vi "Autonomous Independent.vi"() -> ()   [LabVIEW 2020]
doc: "This VI is called when autonomous begins, and will automatically be terminated when autonomous ends. You can carry out timed or sensor driven robot movement independently without needing to return to the caller."
uses:
  <vilib>/Rock Robotics/WPI/RobotDrive/WPI_RobotDriveArcadeDrive_Standard(NoSaturation).vi
  <vilib>/Rock Robotics/Network Tables/NT Write Numeric Array.vi
  <vilib>/Rock Robotics/WPI/ThirdParty/Phoenix-LabVIEW/Motor Controller/Controls/CTRE_Phoenix_MotorControl_ControlMode.ctl
  <vilib>/Rock Robotics/WPI/ThirdParty/Phoenix-LabVIEW/CANCoder/Get/CTRE_Phoenix_CANcoder_GetSensorData.vi
  <vilib>/Rock Robotics/WPI/ThirdParty/Phoenix-LabVIEW/Motor Controller/Get/CTRE_Phoenix_MotorController_GetSelectedSensorData.vi
  <vilib>/Rock Robotics/WPI/Solenoid/WPI_SolenoidValue.ctl
  <vilib>/Rock Robotics/WPI/Solenoid/WPI_SolenoidSetEnum.vi
  <vilib>/Rock Robotics/Network Tables/NT Read String.vi
panel:
  out "Talon Encoder Values 2":i32
  out "Arm Tellescope position":dbl format="%#_13g"
  out "Angle Position":dbl format="%#_13g"
  out "Talon Encoder Values":i32=45
  out "Current Movement, for debugging":T1 {"Y Joystick Value" scale=1.0..-1.0; "X Joystick Value" scale=-1.0..1.0}
  in  "Array of robot movements":T2(array[cluster])=[{"X Joystick Value"=0.39393939393939403, "Y Joystick Value"=0.0, "Delay (sec)"=1.0, "Movement Name"="turn"}, {"X Joystick Value"=-0.3737373737373737, "Y Joystick Value"=0.0, "Delay (sec)"=1.0, "Movement Name"="turn back"}] {"Y Joystick Value" scale=1.0..-1.0; "X Joystick Value" scale=-1.0..1.0}
  # "Be sure to right-click and choose Data Operations>>Make Current Value default if you want to save the array values with the VI"
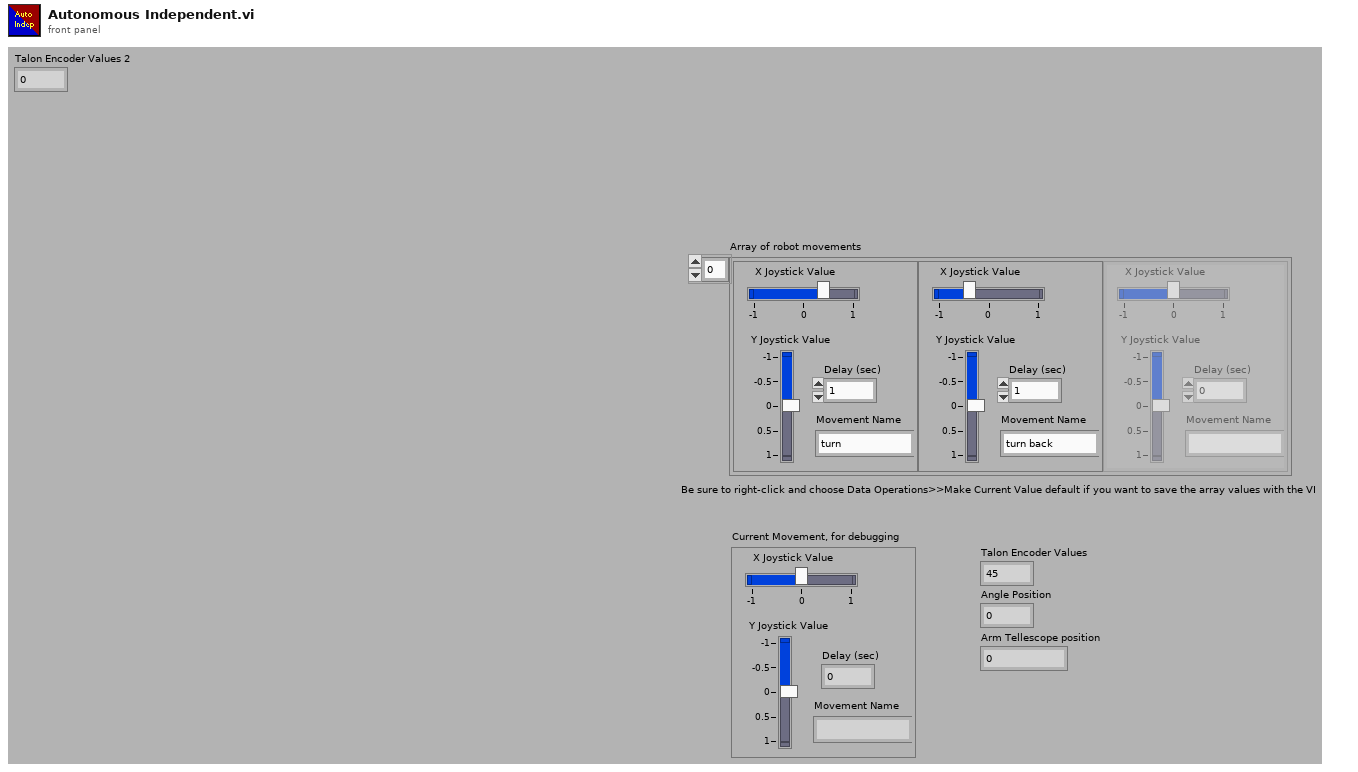
[diagram p1: front panel]
types:
  T1 = cluster{"X Joystick Value":dbl, "Y Joystick Value":dbl, "Delay (sec)":dbl, "Movement Name":string}
  T2 = cluster{"X Joystick Value":dbl, "Y Joystick Value":dbl, "Delay (sec)":dbl, "Movement Name":string}[]
  T3 = typedef "WPI_JoystickDevRef.ctl" = cluster{"Device":T4}
  T4 = typedef "WPI_JoystickDeviceEnum.ctl" = enum16{"USB 0", "USB 1", "USB 2", "USB 3", "USB 4", "USB 5"}
  T5 = typedef "WPI_SolenoidValue.ctl" = enum16{"Off", "On", "Forward", "Reverse"}
  T6 = typedef "WPI_MotorControlDeviceRef.ctl" = cluster{"DeviceStatus":errorcluster, "Type":T7, "PWM":cluster{"PWM Channel":T8, "DeadBand":T9}, "CAN":cluster{"Device Number":u8, "SetOutput VI Ref":variant, "GetOutput VI Ref":variant, "Enable VI Ref":variant, "Disable VI Ref":variant, "Data":variant}, "Invert":bool, "DIO PWM":cluster{"PWM \"Enable\" Channel":T8, "DIOChannel":T10, "PWM Rate":dbl}}
  T7 = typedef "WPI_MotorControlType.ctl" = enum16{"PWM", "CAN", "DIO PWM"}
  T8 = typedef "FPGA_DIOPWMChannel.ctl" = enum8{"PWM 0", "PWM 1", "PWM 2", "PWM 3", "PWM 4", "PWM 5", "PWM 6", "PWM 7", "PWM 8", "PWM 9", "PWM MXP 0", "PWM MXP 1", "PWM MXP 2", "PWM MXP 3", "PWM MXP 4", "PWM MXP 5", "PWM MXP 6", "PWM MXP 7", "PWM MXP 8", "PWM MXP 9", "Invalid"}
  T9 = typedef "WPI_PWMDeadband.ctl" = cluster{"Name":string, "maxPositivePwm":i32, "minPositivePwm":i32, "centerPwm":i32, "maxNegativePwm":i32, "minNegativePwm":i32, "angularRange":u16}
  T10 = typedef "FPGA_DIOChannel.ctl" = enum8{"DIO 0", "DIO 1", "DIO 2", "DIO 3", "DIO 4", "DIO 5", "DIO 6", "DIO 7", "DIO 8", "DIO 9", "DIO MXP 0", "DIO MXP 1", "DIO MXP 2", "DIO MXP 3", "DIO MXP 4", "DIO MXP 5", "DIO MXP 6", "DIO MXP 7", "DIO MXP 8", "DIO MXP 9", "DIO MXP 10", "DIO MXP 11", "DIO MXP 12", "DIO MXP 13", "DIO MXP 14", "DIO MXP 15", "SPI Port CS1", "SPI Port CS2", "SPI Port CS3", "SPI Port MISO", "SPI Port MOSI", "Invalid"}
  T11 = typedef "WPI_RobotDriveDevRef.ctl" = cluster{"DevStatus":errorcluster, "Motors[]":T6[], "Square Inputs":bool, "Max Output":dbl}
  T12 = typedef "CTRE_Phoenix_CANcoder_DeviceRef.ctl" = cluster{"DeviceStatus":errorcluster, "Device Number":u8, "Handle":u64, "UsageFrame":u32, "Library Path":path}
  T13 = typedef "WPI_SolenoidDevRef.ctl" = cluster{"DevStatus":errorcluster, "Pneumatics Control Module":u8, "Forward Solenoid Channel":T14, "Reverse Solenoid Channel":T14}
  T14 = typedef "WPI_SolenoidChannel.ctl" = enum8{"Solenoid 0", "Solenoid 1", "Solenoid 2", "Solenoid 3", "Solenoid 4", "Solenoid 5", "Solenoid 6", "Solenoid 7", "Solenoid 8", "Solenoid 9", "Solenoid 10", "Solenoid 11", "Solenoid 12", "Solenoid 13", "Solenoid 14", "Solenoid 15", "Invalid"}
  T15 = typedef "CTRE_Phoenix_MotorControl_ControlMode.ctl" = u16
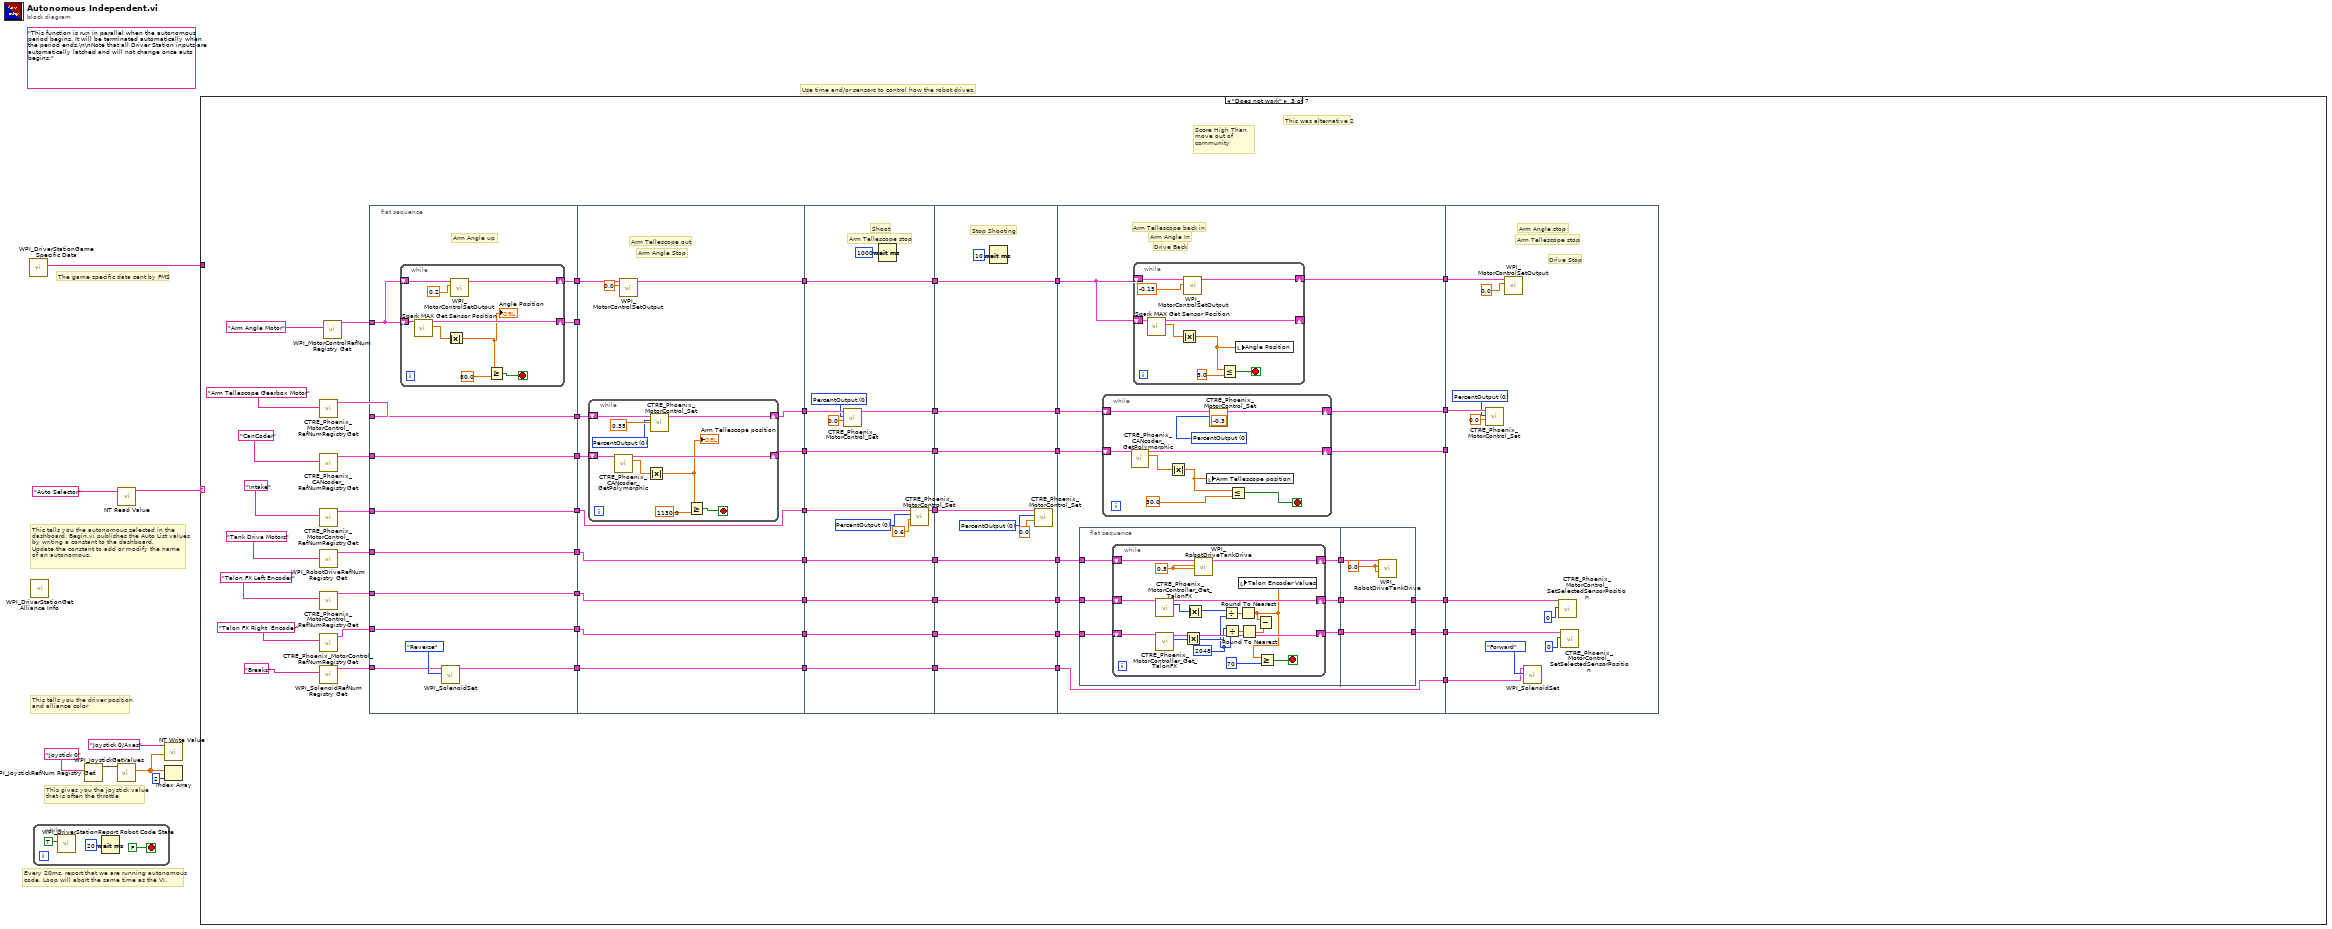
[diagram p0: block diagram]
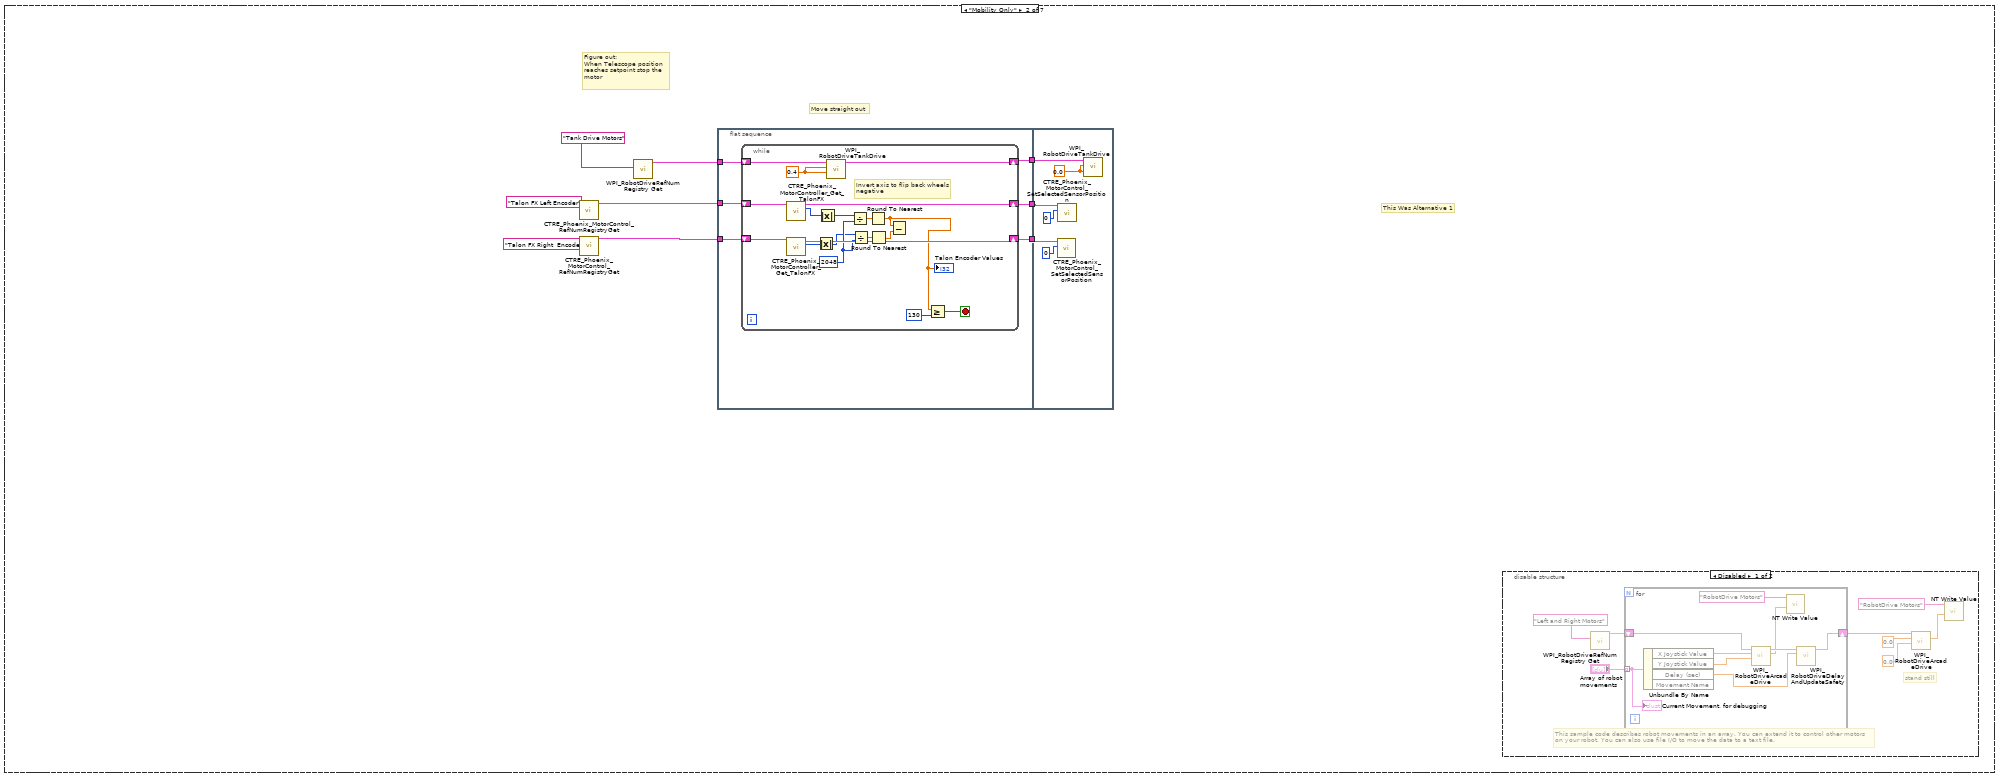
[diagram p3: hidden frame]
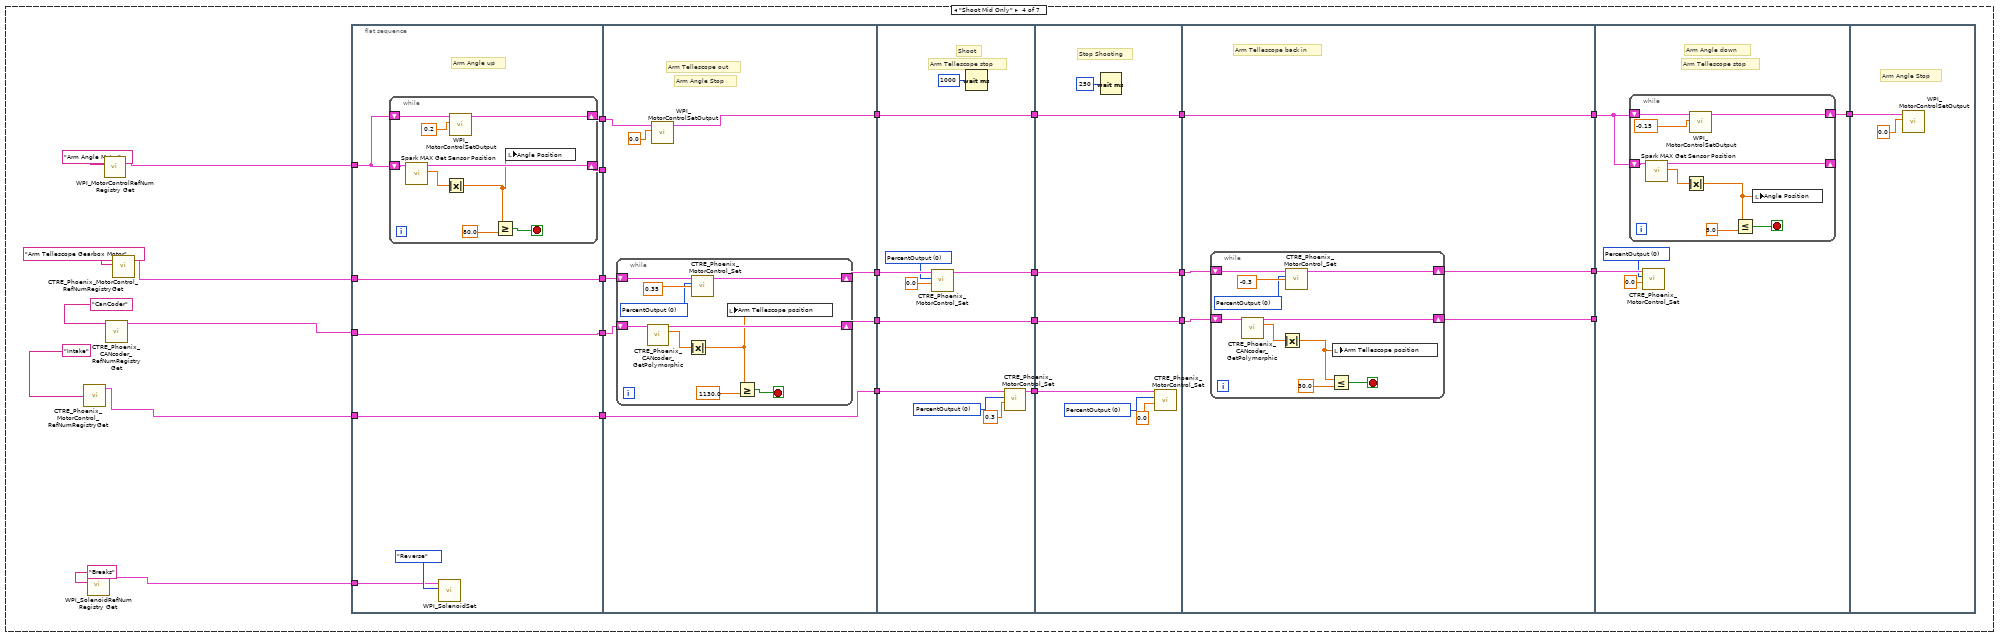
[diagram p5: hidden frame]
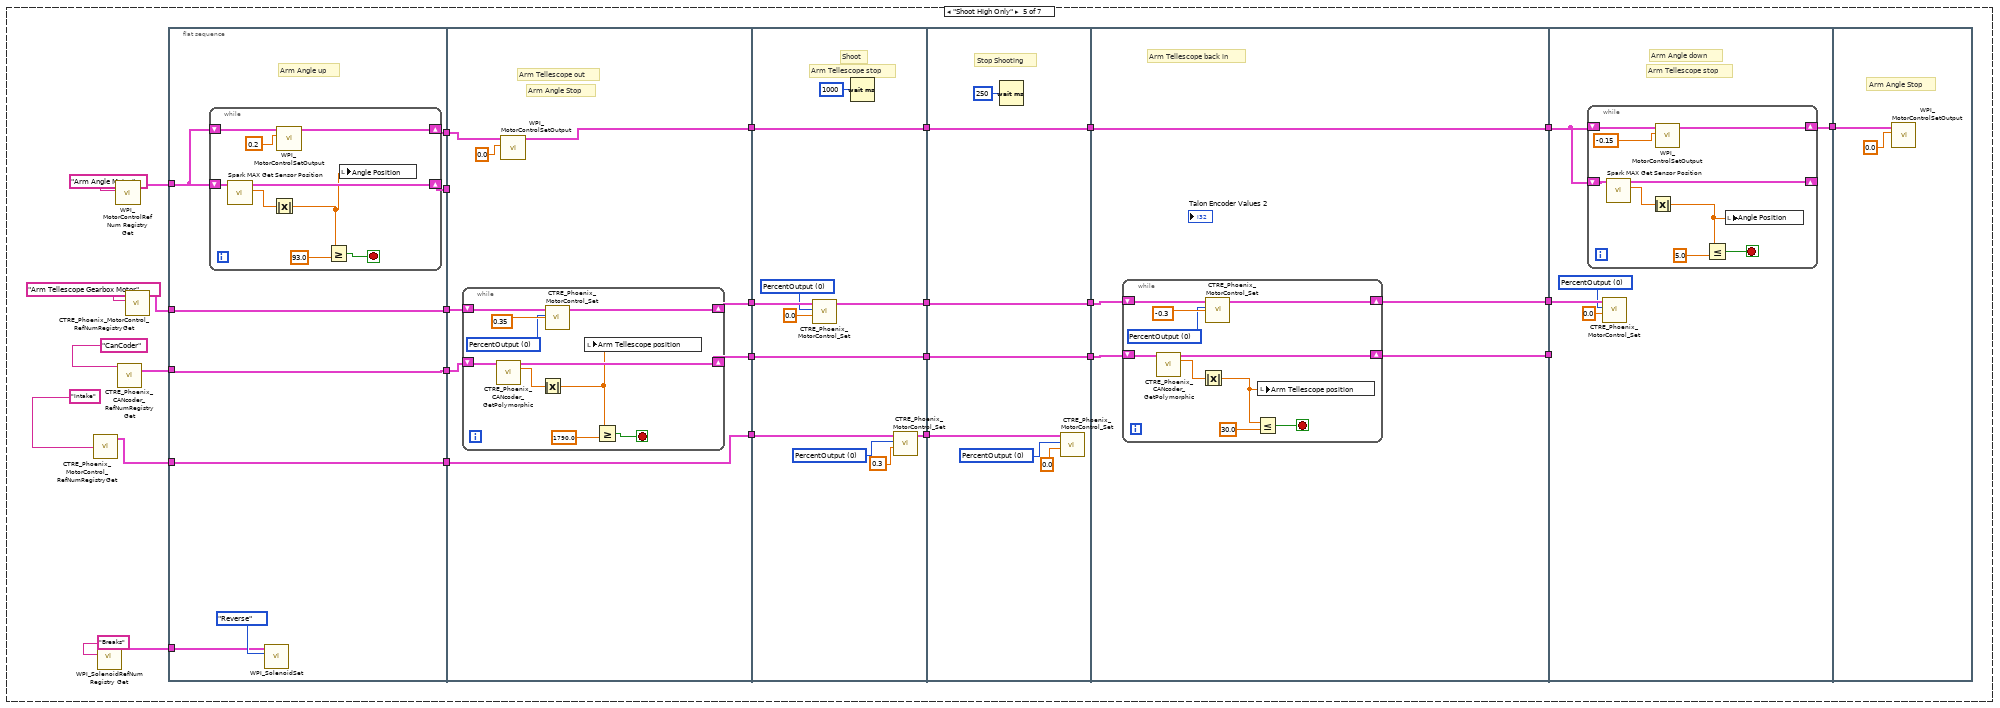
[diagram p6: hidden frame]
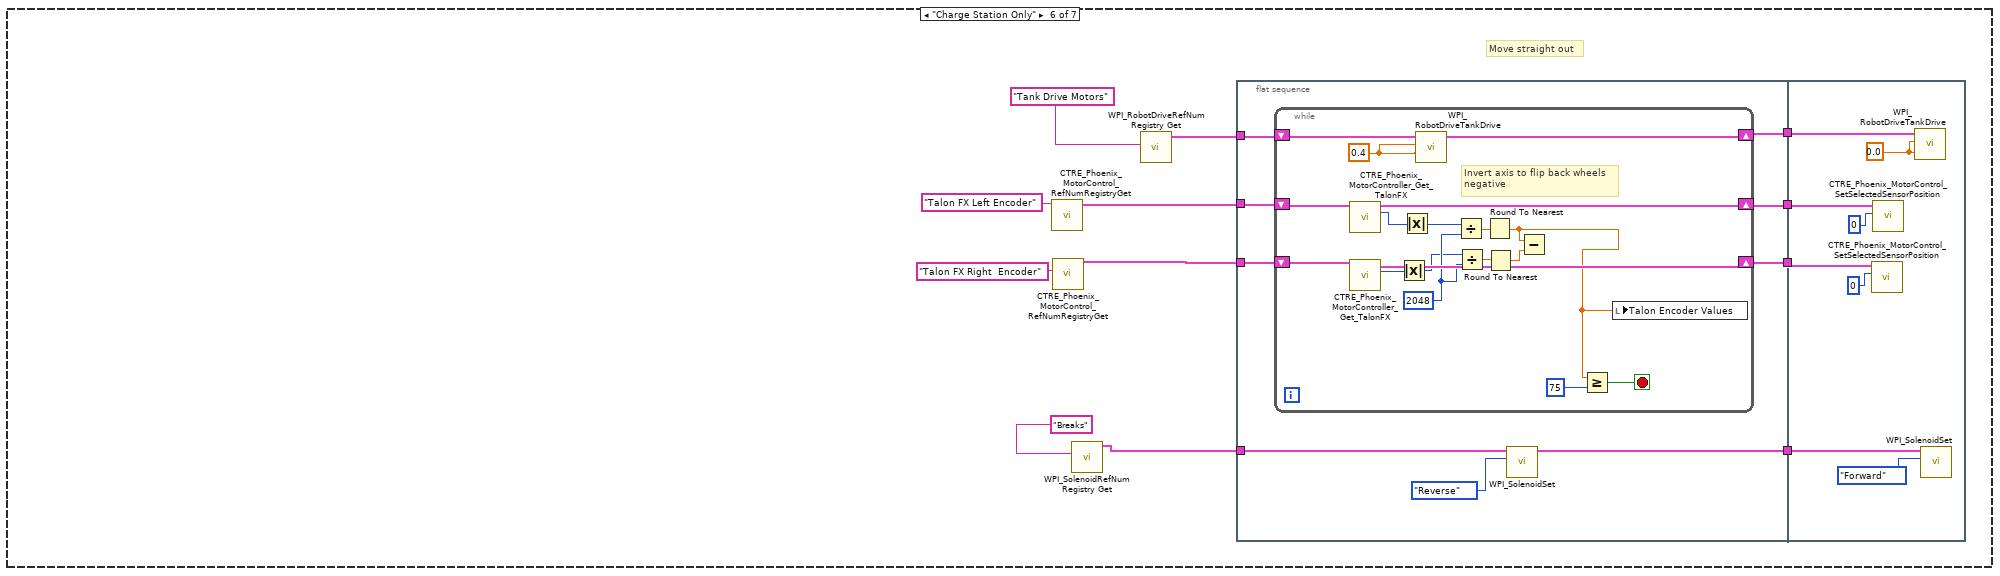
[diagram p7: hidden frame]
diagram:
  (unwired) "This function is run in parallel when the autonomous period begins. It will be terminated automatically when the period ends.\n\nNote that all Driver Station inputs are automatically latched and will not change once auto begins."
  # "The game specific data sent by FMS"
  # "This tells you the autonomous selected in the \ndashboard. Begin.vi publishes the Auto List values\nby writing a constant to the dashboard.\nUpdate the constant to add or modify the name\nof an autonomous."
  # "Every 20ms, report that we are running autonomous\ncode. Loop will abort the same time as the VI."
  # "This gives you the joystick value\nthat is often the throttle"
  # "Use time and/or sensors to control how the robot drives."
  # "This tells you the driver position\nand alliance color"
  n1 = call <vilib>:"WPI_DriverStationGame Specific Data.vi"() -> ("Game Specific Data"=w1:string)  [unwired: 11 in]
  n2 = call <vilib>:"WPI_DriverStationGet Alliance Info.vi"() -> ()  [unwired: 12 out]
  n3 = while {
    stop <- FALSE stop-if-true
    n4 = call <vilib>:"WPI_DriverStationReport Robot Code State.vi"("Autonomous"=TRUE) -> ()  [unwired: 10 in, 1 out]
    n5 = Wait (ms)(milliseconds to wait=u32 20) -> ()  [unwired: 1 out]
  }
  n6 = call <vilib>:"WPI_JoystickRefNum Registry Get.vi"("refnum name"="Joystick 0") -> ("JoystickDevRef"=w7:T3)  [unwired: 1 in, 9 out]
  n7 = call <vilib>:"WPI_JoystickGetValues.vi"("JoystickDevRef"=w7) -> ("Axes"=w3:dbl[])  [unwired: 6 in, 4 out]
  n8 = call-poly <vilib>:"NT Read Value.vi"("name"="Auto Selector" ("Name")) -> ("value"=w4:string)  [unwired: 8 in, 2 out]
  n9 = call-poly <vilib>:"NT Write Value.vi"("value"=w3, "name"="Joystick 0/Axes" ("Name")) -> ()  [unwired: 9 in, 1 out]
  n10 = Index Array(array=w3, index=2) -> ()  [unwired: 1 out]
  n11 = case shown="\"Does not work\"" w4 {
    tunnel: w1 -> [_ _ _ _ _ _ _]
    frame Default {
      # "You can put your main auto here, or you can right-click on the case and make any\nother frame be the default case."
      # "This is the frame that will execute if no selection is made, or if it is not recognized"
    }
    frame "Mobility Only" {
      # "Move straight out"
      # "This Was Alternative 1"
      # "Figure out:\nWhen Telescope position  \nreaches setpoint stop the \nmotor"
      n12 = call <vilib>:"CTRE_Phoenix_MotorControl_RefNumRegistryGet.vi"("refnum name"="Talon FX Left Encoder") -> ("PhoenixMotorControlDevRef"=w12:T6)  [unwired: 9 in, 1 out]
      n13 = call <vilib>:"CTRE_Phoenix_MotorControl_RefNumRegistryGet.vi"("refnum name"="Talon FX Right  Encoder") -> ("PhoenixMotorControlDevRef"=w13:T6)  [unwired: 9 in, 1 out]
      n14 = call <vilib>:"WPI_RobotDriveRefNum Registry Get.vi"("refnum name"="Tank Drive Motors") -> ("RobotDriveDevRef"=w16:T11)  [unwired: 9 in, 1 out]
      n15 = flat-sequence {
        tunnel: w16 -> [w43]
        tunnel: [w42] -> w20
        tunnel: [w41] -> w19
        tunnel: [w40] -> w18
        tunnel: w12 -> [w39]
        tunnel: w13 -> [w38]
        tunnel: w20 -> [w66]
        tunnel: w19 -> [w62]
        tunnel: w18 -> [w65]
        frame #0 {
          n16 = while {
            shift-right: [w58] -> w42
            shift-left: w43 -> [w61]
            shift-right: [w56] -> w41
            shift-left: w39 -> [w59]
            shift-right: [w57] -> w40
            shift-left: w38 -> [w60]
            stop <- w53 stop-if-true
            w50 = 2048 ("y")
            w52 = 0.4 ("Left axis value")
            # "Invert axis to flip back wheels\nnegative"
            n17 = call-poly <vilib>:"CTRE_Phoenix_MotorController_Get_TalonFX.vi"("PhoenixMotorControlDevRef"=w59) -> ("PhoenixMotorControlDevRef"=w56:T6, "Position (Raw Sensor Units)"=w55:i32)  [unwired: 11 in, 2 out]
            n18 = call-poly <vilib>:"CTRE_Phoenix_MotorController_Get_TalonFX.vi"("PhoenixMotorControlDevRef"=w60) -> ("PhoenixMotorControlDevRef"=w57:T6, "Position (Raw Sensor Units)"=w54:i32)  [unwired: 11 in, 2 out]
            n19 = Absolute Value(x=w54) -> (abs(x)=w48:i32)
            n20 = Absolute Value(x=w55) -> (abs(x)=w49:i32)
            n21 = call <vilib>:"WPI_RobotDriveTankDrive.vi"("Right axis value"=w52, "Left axis value"=w52, "RobotDriveDevRef"=w61) -> ("RobotDriveDevRef"=w58:T11)  [unwired: 6 in, 2 out]
            n22 = Divide(x=w49, y=w50) -> (x/y=w47:dbl)
            n23 = Divide(x=w48, y=w50) -> (x/y=w46:dbl)
            n24 = Round To Nearest(number=w47) -> (nearest integer value=w44:dbl)
            "Talon Encoder Values" <- w44
            n25 = Round To Nearest(number=w46) -> (nearest integer value=w45:dbl)
            n26 = Subtract(x=w44, y=w45) -> ()  [unwired: 1 out]
            n27 = Greater Or Equal?(x=w44, y=130) -> (x >= y?=w53:bool)
          }
        }
        frame #1 {
          w67 = 0.0
          n28 = call <vilib>:"CTRE_Phoenix_MotorControl_SetSelectedSensorPosition.vi"("New Sensor Position"=0, "PhoenixMotorControlDevRef"=w65) -> ()  [unwired: 8 in, 2 out]
          n29 = call <vilib>:"CTRE_Phoenix_MotorControl_SetSelectedSensorPosition.vi"("New Sensor Position"=0, "PhoenixMotorControlDevRef"=w62) -> ()  [unwired: 8 in, 2 out]
          n30 = call <vilib>:"WPI_RobotDriveTankDrive.vi"("Right axis value"=w67, "Left axis value"=w67, "RobotDriveDevRef"=w66) -> ()  [unwired: 6 in, 3 out]
        }
      }
      n31 = disable-structure shown="Disabled" {
        frame Disabled {
          # "stand still"
          # "This sample code describes robot movements in an array. You can extend it to control other motors\non your robot. You can also use file I/O to move the data to a text file."
          n32 = call <vilib>:"WPI_RobotDriveRefNum Registry Get.vi"("refnum name"="Left and Right Motors") -> ("RobotDriveDevRef"=w27:T11)  [unwired: 1 in, 9 out]
          n33 = for {
            shift-right: [w35] -> w22
            shift-left: w27 -> [w36]
            tunnel: "Array of robot movements" -> [w31] mode=indexing
            n34 = Unbundle By Name(w31) -> ("X Joystick Value"=w34:dbl, "Y Joystick Value"=w33:dbl, "Delay (sec)"=w32:dbl)  [unwired: 1 out]
            n35 = call-poly <vilib>:"WPI_RobotDriveArcadeDrive.vi"("Y axis value"=w33, "X axis value"=w34, "RobotDriveDevRef"=w36) -> ("Motor Values"=w29:dbl[], "RobotDriveDevRef"=w37:T11)  [unwired: 1 in, 6 out]
            n36 = call-poly <vilib>:"NT Write Value.vi"("value"=w29, "name"="RobotDrive Motors" ("Name")) -> ()  [unwired: 9 in, 1 out]
            n37 = call <vilib>:"WPI_RobotDriveDelayAndUpdateSafety.vi"("Delay (s)"=w32, "RobotDriveDevRef"=w37) -> ("RobotDriveDevRef 2"=w35:T11)  [unwired: 8 in, 1 out]
            "Current Movement, for debugging" <- w31
          }
          n38 = call-poly <vilib>:"WPI_RobotDriveArcadeDrive.vi"("Y axis value"=0.0 ("X axis value"), "X axis value"=0.0, "RobotDriveDevRef"=w22) -> ("Motor Values"=w25:dbl[])  [unwired: 1 in, 7 out]
          n39 = call-poly <vilib>:"NT Write Value.vi"("value"=w25, "name"="RobotDrive Motors" ("Name")) -> ()  [unwired: 9 in, 1 out]
        }
        frame Enabled {
        }
      }
    }
    frame "Does not work" {
      # "This was alternative 2"
      # "Score High Than \nmove out of \ncommunity"
      n40 = call <vilib>:"CTRE_Phoenix_MotorControl_RefNumRegistryGet.vi"("refnum name"="Arm Tellescope Gearbox Motor") -> ("PhoenixMotorControlDevRef"=w93:T6)  [unwired: 9 in, 1 out]
      n41 = call <vilib>:"CTRE_Phoenix_CANcoder_RefNumRegistryGet.vi"("refnum name"="CanCoder") -> ("CTRE_CANcoder_DeviceRef"=w97:T12)  [unwired: 9 in, 1 out]
      n42 = call <vilib>:"CTRE_Phoenix_MotorControl_RefNumRegistryGet.vi"("refnum name"="Intake") -> ("PhoenixMotorControlDevRef"=w107:T6)  [unwired: 9 in, 1 out]
      n43 = call <vilib>:"WPI_RobotDriveRefNum Registry Get.vi"("refnum name"="Tank Drive Motors") -> ("RobotDriveDevRef"=w77:T11)  [unwired: 9 in, 1 out]
      n44 = call <vilib>:"CTRE_Phoenix_MotorControl_RefNumRegistryGet.vi"("refnum name"="Talon FX Left Encoder") -> ("PhoenixMotorControlDevRef"=w82:T6)  [unwired: 9 in, 1 out]
      n45 = call <vilib>:"CTRE_Phoenix_MotorControl_RefNumRegistryGet.vi"("refnum name"="Talon FX Right  Encoder") -> ("PhoenixMotorControlDevRef"=w87:T6)  [unwired: 9 in, 1 out]
      n46 = call <vilib>:"WPI_SolenoidRefNum Registry Get.vi"("refnum name"="Breaks") -> ("SolenoidDevRef"=w101:T13)  [unwired: 9 in, 1 out]
      n47 = call <vilib>:"WPI_MotorControlRefNum Registry Get.vi"("refnum name"="Arm Angle Motor") -> ("MotorControlDevRef"=w109:T6)  [unwired: 9 in, 1 out]
      n48 = flat-sequence {
        tunnel: w109 -> [w132]
        tunnel: [w133] -> w121
        tunnel: w107 -> [w133]
        tunnel: w101 -> [w130]
        tunnel: [w129] -> w100
        tunnel: [w128] -> w99
        tunnel: w97 -> [w127]
        tunnel: [w127] -> w98
        tunnel: [w126] -> w94
        tunnel: w93 -> [w126]
        tunnel: [w125] -> w88
        tunnel: w87 -> [w125]
        tunnel: [w124] -> w83
        tunnel: w82 -> [w124]
        tunnel: [w123] -> w78
        tunnel: w77 -> [w123]
        tunnel: [w122] -> w72
        tunnel: w121 -> [w154]
        tunnel: [w154] -> w120
        tunnel: [w148] -> w119
        tunnel: [w153] -> w118
        tunnel: [w152] -> w117
        tunnel: w100 -> [w149]
        tunnel: w99 -> [_]
        tunnel: w98 -> [w151]
        tunnel: w94 -> [w150]
        tunnel: w88 -> [w146]
        tunnel: [w146] -> w84
        tunnel: w83 -> [w145]
        tunnel: [w145] -> w79
        tunnel: w78 -> [w144]
        tunnel: [w144] -> w74
        tunnel: w72 -> [w143]
        tunnel: [w143] -> w71
        tunnel: w120 -> [w177]
        tunnel: [w175] -> w116
        tunnel: w119 -> [w174]
        tunnel: [w174] -> w115
        tunnel: [w171] -> w114
        tunnel: w118 -> [w172]
        tunnel: [w173] -> w113
        tunnel: w117 -> [w173]
        tunnel: [w168] -> w85
        tunnel: w84 -> [w168]
        tunnel: [w167] -> w80
        tunnel: w79 -> [w167]
        tunnel: [w166] -> w75
        tunnel: w74 -> [w166]
        tunnel: w71 -> [w165]
        tunnel: [w165] -> w70
        tunnel: w116 -> [w188]
        tunnel: w115 -> [w186]
        tunnel: [w186] -> w112
        tunnel: [w185] -> w111
        tunnel: w114 -> [w185]
        tunnel: [w184] -> w110
        tunnel: w113 -> [w184]
        tunnel: [w183] -> w86
        tunnel: w85 -> [w183]
        tunnel: [w182] -> w81
        tunnel: w80 -> [w182]
        tunnel: [w181] -> w76
        tunnel: w75 -> [w181]
        tunnel: w70 -> [w180]
        tunnel: [w180] -> w69
        tunnel: w112 -> [w203]
        tunnel: w111 -> [w205]
        tunnel: w110 -> [w204]
        tunnel: [w202] -> w92
        tunnel: [w201] -> w91
        tunnel: [w200] -> w90
        tunnel: [w199] -> w89
        tunnel: w86 -> [w198]
        tunnel: w81 -> [w197]
        tunnel: w76 -> [w196]
        tunnel: [w195] -> w73
        tunnel: w69 -> [w194]
        tunnel: [w194] -> w68
        tunnel: w92 -> [w263]
        tunnel: w91 -> [_]
        tunnel: w90 -> [w258]
        tunnel: w89 -> [w257]
        tunnel: w73 -> [w256]
        tunnel: w68 -> [w253]
        frame #0 {
          # "Arm Angle up"
          n49 = while {
            shift-right: [w136] -> w129
            shift-left: w132 -> [w135]
            shift-right: [w139] -> w128
            shift-left: w132 -> [w140]
            stop <- w142 stop-if-true
            n50 = call <vilib>:"Spark MAX Get Sensor Position.vi"("MotorControlDevRef in"=w140) -> ("Sensor Position"=w138:dbl, "MotorControlDevRef out"=w139:T6)  [unwired: 7 in, 2 out]
            n51 = Absolute Value(x=w138) -> (abs(x)=w134:dbl)
            "Angle Position" <- w134
            n52 = call <vilib>:"WPI_MotorControlSetOutput.vi"("Output"=0.2 ("Left axis value"), "MotorControlDevRef"=w135) -> ("MotorControlDevRef"=w136:T6)  [unwired: 7 in, 2 out]
            n53 = Greater Or Equal?(x=w134, y=80.0) -> (x >= y?=w142:bool)
          }
          n54 = call-poly <vilib>:"WPI_SolenoidSet.vi"("Value"=WPI_SolenoidValue."Reverse", "SolenoidDevRef"=w130) -> ("SolenoidDevRef"=w122:T13)  [unwired: 8 in, 1 out]
        }
        frame #1 {
          # "Arm Angle Stop"
          # "Arm Tellescope out"
          n55 = while {
            shift-right: [w158] -> w153
            shift-left: w150 -> [w157]
            shift-right: [w161] -> w152
            shift-left: w151 -> [w162]
            stop <- w164 stop-if-true
            w156 = T15 0 items=["PercentOutput"=0, "Position"=1, "Velocity"=2, "Current"=3, "Follower"=5, "MotionProfile"=6, "MotionMagic"=7, "MotionProfileArc"=10, "Disabled"=15] ("Control Mode")
            n56 = call-poly <vilib>:"CTRE_Phoenix_CANcoder_GetPolymorphic.vi"("CTRE_CANcoder_DeviceRef"=w162) -> ("CTRE_CANcoder_DeviceRef"=w161:T12, "Position"=w160:dbl)  [unwired: 10 in, 3 out]
            n57 = Absolute Value(x=w160) -> (abs(x)=w155:dbl)
            "Arm Tellescope position" <- w155
            n58 = call <vilib>:"CTRE_Phoenix_MotorControl_Set.vi"("Output"=0.35 ("Left axis value"), "Control Mode"=w156, "PhoenixMotorControlDevRef"=w157) -> ("PhoenixMotorControlDevRef"=w158:T6)  [unwired: 7 in, 1 out]
            n59 = Greater Or Equal?(x=w155, y=1130.0) -> (x >= y?=w164:bool)
          }
          n60 = call <vilib>:"WPI_MotorControlSetOutput.vi"("Output"=0.0, "MotorControlDevRef"=w149) -> ("MotorControlDevRef"=w148:T6)  [unwired: 7 in, 2 out]
        }
        frame #2 {
          w170 = T15 0 items=["PercentOutput"=0, "Position"=1, "Velocity"=2, "Current"=3, "Follower"=5, "MotionProfile"=6, "MotionMagic"=7, "MotionProfileArc"=10, "Disabled"=15] ("Control Mode")
          w179 = T15 0 items=["PercentOutput"=0, "Position"=1, "Velocity"=2, "Current"=3, "Follower"=5, "MotionProfile"=6, "MotionMagic"=7, "MotionProfileArc"=10, "Disabled"=15] ("Control Mode")
          # "Arm Tellescope stop"
          # "Shoot"
          n61 = call <vilib>:"CTRE_Phoenix_MotorControl_Set.vi"("Output"=0.0, "Control Mode"=w170, "PhoenixMotorControlDevRef"=w172) -> ("PhoenixMotorControlDevRef"=w171:T6)  [unwired: 7 in, 1 out]
          n62 = Wait (ms)(milliseconds to wait=u32 1000) -> ()  [unwired: 1 out]
          n63 = call <vilib>:"CTRE_Phoenix_MotorControl_Set.vi"("Output"=0.6, "Control Mode"=w179, "PhoenixMotorControlDevRef"=w177) -> ("PhoenixMotorControlDevRef"=w175:T6)  [unwired: 7 in, 1 out]
        }
        frame #3 {
          w189 = T15 0 items=["PercentOutput"=0, "Position"=1, "Velocity"=2, "Current"=3, "Follower"=5, "MotionProfile"=6, "MotionMagic"=7, "MotionProfileArc"=10, "Disabled"=15] ("Control Mode")
          # "Stop Shooting"
          n64 = Wait (ms)(milliseconds to wait=u32 10) -> ()  [unwired: 1 out]
          n65 = call <vilib>:"CTRE_Phoenix_MotorControl_Set.vi"("Output"=0.0, "Control Mode"=w189, "PhoenixMotorControlDevRef"=w188) -> ()  [unwired: 7 in, 2 out]
        }
        frame #4 {
          # "Drive Back"
          # "Arm Angle In"
          # "Arm Tellescope back in"
          n66 = flat-sequence {
            tunnel: w198 -> [w208]
            tunnel: w197 -> [w207]
            tunnel: w196 -> [w206]
            tunnel: [w211] -> w193
            tunnel: [w210] -> w192
            tunnel: [w209] -> w191
            tunnel: [w232] -> w199
            tunnel: [w233] -> w200
            tunnel: w193 -> [w231]
            tunnel: w192 -> [w233]
            tunnel: w191 -> [w232]
            frame #0 {
              n67 = while {
                shift-right: [w226] -> w211
                shift-left: w206 -> [w229]
                shift-right: [w224] -> w210
                shift-left: w207 -> [w227]
                shift-right: [w225] -> w209
                shift-left: w208 -> [w228]
                stop <- w221 stop-if-true
                w215 = 2048
                w220 = 0.5 ("Left axis value")
                n68 = call-poly <vilib>:"CTRE_Phoenix_MotorController_Get_TalonFX.vi"("PhoenixMotorControlDevRef"=w227) -> ("PhoenixMotorControlDevRef"=w224:T6, "Position (Raw Sensor Units)"=w223:i32)  [unwired: 11 in, 2 out]
                n69 = call-poly <vilib>:"CTRE_Phoenix_MotorController_Get_TalonFX.vi"("PhoenixMotorControlDevRef"=w228) -> ("PhoenixMotorControlDevRef"=w225:T6, "Position (Raw Sensor Units)"=w222:i32)  [unwired: 11 in, 2 out]
                n70 = Absolute Value(x=w222) -> (abs(x)=w216:i32)
                n71 = Absolute Value(x=w223) -> (abs(x)=w214:i32)
                n72 = call <vilib>:"WPI_RobotDriveTankDrive.vi"("Right axis value"=w220, "Left axis value"=w220, "RobotDriveDevRef"=w229) -> ("RobotDriveDevRef"=w226:T11)  [unwired: 6 in, 2 out]
                n73 = Divide(x=w214, y=w215) -> (x/y=w217:dbl)
                n74 = Divide(x=w216, y=w215) -> (x/y=w218:dbl)
                n75 = Round To Nearest(number=w217) -> (nearest integer value=w212:dbl)
                n76 = local write "Talon Encoder Values"(w212) -> ()
                n77 = Round To Nearest(number=w218) -> (nearest integer value=w213:dbl)
                n78 = Subtract(x=w212, y=w213) -> ()  [unwired: 1 out]
                n79 = Greater Or Equal?(x=w212, y=70) -> (x >= y?=w221:bool)
              }
            }
            frame #1 {
              w230 = 0.0 ("Left axis value")
              n80 = call <vilib>:"WPI_RobotDriveTankDrive.vi"("Right axis value"=w230, "Left axis value"=w230, "RobotDriveDevRef"=w231) -> ()  [unwired: 6 in, 3 out]
            }
          }
          n81 = while {
            shift-right: [w246] -> w202
            shift-left: w205 -> [w245]
            shift-right: [w249] -> w201
            shift-left: w204 -> [w250]
            stop <- w252 stop-if-true
            w244 = T15 0 items=["PercentOutput"=0, "Position"=1, "Velocity"=2, "Current"=3, "Follower"=5, "MotionProfile"=6, "MotionMagic"=7, "MotionProfileArc"=10, "Disabled"=15] ("Control Mode")
            n82 = call-poly <vilib>:"CTRE_Phoenix_CANcoder_GetPolymorphic.vi"("CTRE_CANcoder_DeviceRef"=w250) -> ("CTRE_CANcoder_DeviceRef"=w249:T12, "Position"=w248:dbl)  [unwired: 10 in, 3 out]
            n83 = Absolute Value(x=w248) -> (abs(x)=w243:dbl)
            n84 = local write "Arm Tellescope position"(w243) -> ()
            n85 = call <vilib>:"CTRE_Phoenix_MotorControl_Set.vi"("Output"=-0.3 ("Left axis value"), "Control Mode"=w244, "PhoenixMotorControlDevRef"=w245) -> ("PhoenixMotorControlDevRef"=w246:T6)  [unwired: 7 in, 1 out]
            n86 = Less Or Equal?(x=w243, y=30.0) -> (x <= y?=w252:bool)
          }
          n87 = while {
            shift-right: [w237] -> w195
            shift-left: w203 -> [w236]
            shift-right: [w239] -> _
            shift-left: w203 -> [w240]
            stop <- w242 stop-if-true
            n88 = call <vilib>:"Spark MAX Get Sensor Position.vi"("MotorControlDevRef in"=w240) -> ("Sensor Position"=w238:dbl, "MotorControlDevRef out"=w239:T6)  [unwired: 7 in, 2 out]
            n89 = Absolute Value(x=w238) -> (abs(x)=w234:dbl)
            n90 = call <vilib>:"WPI_MotorControlSetOutput.vi"("Output"=-0.15 ("Left axis value"), "MotorControlDevRef"=w236) -> ("MotorControlDevRef"=w237:T6)  [unwired: 7 in, 2 out]
            n91 = Less Or Equal?(x=w234, y=5.0) -> (x <= y?=w242:bool)
            n92 = local write "Angle Position"(w234) -> ()
          }
        }
        frame #5 {
          w261 = T15 0 items=["PercentOutput"=0, "Position"=1, "Velocity"=2, "Current"=3, "Follower"=5, "MotionProfile"=6, "MotionMagic"=7, "MotionProfileArc"=10, "Disabled"=15] ("Control Mode")
          # "Drive Stop"
          # "Arm Tellescope stop"
          # "Arm Angle stop"
          n93 = call <vilib>:"CTRE_Phoenix_MotorControl_Set.vi"("Output"=0.0, "Control Mode"=w261, "PhoenixMotorControlDevRef"=w263) -> ()  [unwired: 7 in, 2 out]
          n94 = call <vilib>:"WPI_MotorControlSetOutput.vi"("Output"=0.0, "MotorControlDevRef"=w256) -> ()  [unwired: 7 in, 3 out]
          n95 = call-poly <vilib>:"WPI_SolenoidSet.vi"("Value"=WPI_SolenoidValue."Forward", "SolenoidDevRef"=w253) -> ()  [unwired: 8 in, 2 out]
          n96 = call <vilib>:"CTRE_Phoenix_MotorControl_SetSelectedSensorPosition.vi"("New Sensor Position"=0, "PhoenixMotorControlDevRef"=w258) -> ()  [unwired: 8 in, 2 out]
          n97 = call <vilib>:"CTRE_Phoenix_MotorControl_SetSelectedSensorPosition.vi"("New Sensor Position"=0, "PhoenixMotorControlDevRef"=w257) -> ()  [unwired: 8 in, 2 out]
        }
      }
    }
    frame "Shoot Mid Only" {
      n98 = call <vilib>:"CTRE_Phoenix_MotorControl_RefNumRegistryGet.vi"("refnum name"="Intake") -> ("PhoenixMotorControlDevRef"=w266:T6)  [unwired: 9 in, 1 out]
      n99 = call <vilib>:"WPI_SolenoidRefNum Registry Get.vi"("refnum name"="Breaks") -> ("SolenoidDevRef"=w265:T13)  [unwired: 9 in, 1 out]
      n100 = call <vilib>:"WPI_MotorControlRefNum Registry Get.vi"("refnum name"="Arm Angle Motor") -> ("MotorControlDevRef"=w264:T6)  [unwired: 9 in, 1 out]
      n101 = call <vilib>:"CTRE_Phoenix_CANcoder_RefNumRegistryGet.vi"("refnum name"="CanCoder") -> ("CTRE_CANcoder_DeviceRef"=w267:T12)  [unwired: 9 in, 1 out]
      n102 = call <vilib>:"CTRE_Phoenix_MotorControl_RefNumRegistryGet.vi"("refnum name"="Arm Tellescope Gearbox Motor") -> ("PhoenixMotorControlDevRef"=w268:T6)  [unwired: 9 in, 1 out]
      n103 = flat-sequence {
        tunnel: w264 -> [w301]
        tunnel: [w299] -> w293
        tunnel: [w298] -> w292
        tunnel: [w297] -> w291
        tunnel: w267 -> [w297]
        tunnel: w265 -> [w296]
        tunnel: [w295] -> w290
        tunnel: w268 -> [w295]
        tunnel: [w294] -> w289
        tunnel: w266 -> [w294]
        tunnel: [w315] -> w288
        tunnel: [w318] -> w287
        tunnel: [w317] -> w286
        tunnel: w293 -> [w316]
        tunnel: w292 -> [_]
        tunnel: w291 -> [w313]
        tunnel: w290 -> [w312]
        tunnel: w289 -> [w311]
        tunnel: [w311] -> w285
        tunnel: [w336] -> w284
        tunnel: w288 -> [w335]
        tunnel: [w335] -> w283
        tunnel: [w332] -> w282
        tunnel: w287 -> [w333]
        tunnel: [w334] -> w281
        tunnel: w286 -> [w334]
        tunnel: w285 -> [w329]
        tunnel: w284 -> [w344]
        tunnel: w283 -> [w342]
        tunnel: [w342] -> w280
        tunnel: [w341] -> w279
        tunnel: w282 -> [w341]
        tunnel: [w340] -> w278
        tunnel: w281 -> [w340]
        tunnel: w280 -> [w349]
        tunnel: w279 -> [w351]
        tunnel: w278 -> [w350]
        tunnel: [w349] -> w277
        tunnel: [w348] -> w276
        tunnel: [w347] -> w275
        tunnel: w277 -> [w366]
        tunnel: w276 -> [w365]
        tunnel: w275 -> [_]
        tunnel: [w362] -> w274
        tunnel: w274 -> [w377]
        frame #0 {
          # "Arm Angle up"
          n104 = while {
            shift-right: [w304] -> w299
            shift-left: w301 -> [w303]
            shift-right: [w307] -> w298
            shift-left: w301 -> [w308]
            stop <- w310 stop-if-true
            n105 = call <vilib>:"Spark MAX Get Sensor Position.vi"("MotorControlDevRef in"=w308) -> ("Sensor Position"=w306:dbl, "MotorControlDevRef out"=w307:T6)  [unwired: 7 in, 2 out]
            n106 = Absolute Value(x=w306) -> (abs(x)=w302:dbl)
            n107 = call <vilib>:"WPI_MotorControlSetOutput.vi"("Output"=0.2 ("Left axis value"), "MotorControlDevRef"=w303) -> ("MotorControlDevRef"=w304:T6)  [unwired: 7 in, 2 out]
            n108 = Greater Or Equal?(x=w302, y=80.0) -> (x >= y?=w310:bool)
            n109 = local write "Angle Position"(w302) -> ()
          }
          n110 = call-poly <vilib>:"WPI_SolenoidSet.vi"("Value"=WPI_SolenoidValue."Reverse", "SolenoidDevRef"=w296) -> ()  [unwired: 8 in, 2 out]
        }
        frame #1 {
          # "Arm Angle Stop"
          # "Arm Tellescope out"
          n111 = while {
            shift-right: [w322] -> w318
            shift-left: w312 -> [w321]
            shift-right: [w325] -> w317
            shift-left: w313 -> [w326]
            stop <- w328 stop-if-true
            w320 = T15 0 items=["PercentOutput"=0, "Position"=1, "Velocity"=2, "Current"=3, "Follower"=5, "MotionProfile"=6, "MotionMagic"=7, "MotionProfileArc"=10, "Disabled"=15] ("Control Mode")
            n112 = call-poly <vilib>:"CTRE_Phoenix_CANcoder_GetPolymorphic.vi"("CTRE_CANcoder_DeviceRef"=w326) -> ("CTRE_CANcoder_DeviceRef"=w325:T12, "Position"=w324:dbl)  [unwired: 10 in, 3 out]
            n113 = Absolute Value(x=w324) -> (abs(x)=w319:dbl)
            n114 = call <vilib>:"CTRE_Phoenix_MotorControl_Set.vi"("Output"=0.35 ("Left axis value"), "Control Mode"=w320, "PhoenixMotorControlDevRef"=w321) -> ("PhoenixMotorControlDevRef"=w322:T6)  [unwired: 7 in, 1 out]
            n115 = local write "Arm Tellescope position"(w319) -> ()
            n116 = Greater Or Equal?(x=w319, y=1130.0) -> (x >= y?=w328:bool)
          }
          n117 = call <vilib>:"WPI_MotorControlSetOutput.vi"("Output"=0.0, "MotorControlDevRef"=w316) -> ("MotorControlDevRef"=w315:T6)  [unwired: 7 in, 2 out]
        }
        frame #2 {
          w331 = T15 0 items=["PercentOutput"=0, "Position"=1, "Velocity"=2, "Current"=3, "Follower"=5, "MotionProfile"=6, "MotionMagic"=7, "MotionProfileArc"=10, "Disabled"=15] ("Control Mode")
          w339 = T15 0 items=["PercentOutput"=0, "Position"=1, "Velocity"=2, "Current"=3, "Follower"=5, "MotionProfile"=6, "MotionMagic"=7, "MotionProfileArc"=10, "Disabled"=15] ("Control Mode")
          # "Arm Tellescope stop"
          # "Shoot"
          n118 = call <vilib>:"CTRE_Phoenix_MotorControl_Set.vi"("Output"=0.0, "Control Mode"=w331, "PhoenixMotorControlDevRef"=w333) -> ("PhoenixMotorControlDevRef"=w332:T6)  [unwired: 7 in, 1 out]
          n119 = Wait (ms)(milliseconds to wait=u32 1000) -> ()  [unwired: 1 out]
          n120 = call <vilib>:"CTRE_Phoenix_MotorControl_Set.vi"("Output"=0.3, "Control Mode"=w339, "PhoenixMotorControlDevRef"=w329) -> ("PhoenixMotorControlDevRef"=w336:T6)  [unwired: 7 in, 1 out]
        }
        frame #3 {
          w345 = T15 0 items=["PercentOutput"=0, "Position"=1, "Velocity"=2, "Current"=3, "Follower"=5, "MotionProfile"=6, "MotionMagic"=7, "MotionProfileArc"=10, "Disabled"=15] ("Control Mode")
          # "Stop Shooting"
          n121 = Wait (ms)(milliseconds to wait=u32 250) -> ()  [unwired: 1 out]
          n122 = call <vilib>:"CTRE_Phoenix_MotorControl_Set.vi"("Output"=0.0, "Control Mode"=w345, "PhoenixMotorControlDevRef"=w344) -> ()  [unwired: 7 in, 2 out]
        }
        frame #4 {
          # "Arm Tellescope back in"
          n123 = while {
            shift-right: [w355] -> w348
            shift-left: w351 -> [w354]
            shift-right: [w358] -> w347
            shift-left: w350 -> [w359]
            stop <- w361 stop-if-true
            w353 = T15 0 items=["PercentOutput"=0, "Position"=1, "Velocity"=2, "Current"=3, "Follower"=5, "MotionProfile"=6, "MotionMagic"=7, "MotionProfileArc"=10, "Disabled"=15] ("Control Mode")
            n124 = call-poly <vilib>:"CTRE_Phoenix_CANcoder_GetPolymorphic.vi"("CTRE_CANcoder_DeviceRef"=w359) -> ("CTRE_CANcoder_DeviceRef"=w358:T12, "Position"=w357:dbl)  [unwired: 10 in, 3 out]
            n125 = Absolute Value(x=w357) -> (abs(x)=w352:dbl)
            n126 = call <vilib>:"CTRE_Phoenix_MotorControl_Set.vi"("Output"=-0.3 ("Left axis value"), "Control Mode"=w353, "PhoenixMotorControlDevRef"=w354) -> ("PhoenixMotorControlDevRef"=w355:T6)  [unwired: 7 in, 1 out]
            n127 = Less Or Equal?(x=w352, y=30.0) -> (x <= y?=w361:bool)
            n128 = local write "Arm Tellescope position"(w352) -> ()
          }
        }
        frame #5 {
          w363 = T15 0 items=["PercentOutput"=0, "Position"=1, "Velocity"=2, "Current"=3, "Follower"=5, "MotionProfile"=6, "MotionMagic"=7, "MotionProfileArc"=10, "Disabled"=15] ("Control Mode")
          # "Arm Tellescope stop"
          # "Arm Angle down"
          n129 = while {
            shift-right: [w370] -> w362
            shift-left: w366 -> [w369]
            shift-right: [w372] -> _
            shift-left: w366 -> [w373]
            stop <- w375 stop-if-true
            n130 = call <vilib>:"Spark MAX Get Sensor Position.vi"("MotorControlDevRef in"=w373) -> ("Sensor Position"=w371:dbl, "MotorControlDevRef out"=w372:T6)  [unwired: 7 in, 2 out]
            n131 = Absolute Value(x=w371) -> (abs(x)=w367:dbl)
            n132 = call <vilib>:"WPI_MotorControlSetOutput.vi"("Output"=-0.15 ("Left axis value"), "MotorControlDevRef"=w369) -> ("MotorControlDevRef"=w370:T6)  [unwired: 7 in, 2 out]
            n133 = Less Or Equal?(x=w367, y=5.0) -> (x <= y?=w375:bool)
            n134 = local write "Angle Position"(w367) -> ()
          }
          n135 = call <vilib>:"CTRE_Phoenix_MotorControl_Set.vi"("Output"=0.0, "Control Mode"=w363, "PhoenixMotorControlDevRef"=w365) -> ()  [unwired: 7 in, 2 out]
        }
        frame #6 {
          # "Arm Angle Stop"
          n136 = call <vilib>:"WPI_MotorControlSetOutput.vi"("Output"=0.0, "MotorControlDevRef"=w377) -> ()  [unwired: 7 in, 3 out]
        }
      }
    }
    frame "Shoot High Only" {
      n137 = call <vilib>:"CTRE_Phoenix_MotorControl_RefNumRegistryGet.vi"("refnum name"="Intake") -> ("PhoenixMotorControlDevRef"=w379:T6)  [unwired: 9 in, 1 out]
      n138 = call <vilib>:"WPI_SolenoidRefNum Registry Get.vi"("refnum name"="Breaks") -> ("SolenoidDevRef"=w384:T13)  [unwired: 9 in, 1 out]
      n139 = call <vilib>:"WPI_MotorControlRefNum Registry Get.vi"("refnum name"="Arm Angle Motor") -> ("MotorControlDevRef"=w388:T6)  [unwired: 9 in, 1 out]
      n140 = call <vilib>:"CTRE_Phoenix_CANcoder_RefNumRegistryGet.vi"("refnum name"="CanCoder") -> ("CTRE_CANcoder_DeviceRef"=w386:T12)  [unwired: 9 in, 1 out]
      n141 = call <vilib>:"CTRE_Phoenix_MotorControl_RefNumRegistryGet.vi"("refnum name"="Arm Tellescope Gearbox Motor") -> ("PhoenixMotorControlDevRef"=w382:T6)  [unwired: 9 in, 1 out]
      n142 = flat-sequence {
        tunnel: w388 -> [w415]
        tunnel: [w413] -> w407
        tunnel: [w412] -> w406
        tunnel: [w411] -> w387
        tunnel: w386 -> [w411]
        tunnel: w384 -> [w410]
        tunnel: [w409] -> w383
        tunnel: w382 -> [w409]
        tunnel: [w408] -> w380
        tunnel: w379 -> [w408]
        tunnel: [w429] -> w405
        tunnel: [w432] -> w404
        tunnel: [w431] -> w403
        tunnel: w407 -> [w430]
        tunnel: w406 -> [_]
        tunnel: w387 -> [w427]
        tunnel: w383 -> [w426]
        tunnel: w380 -> [w425]
        tunnel: [w425] -> w378
        tunnel: [w450] -> w402
        tunnel: w405 -> [w449]
        tunnel: [w449] -> w401
        tunnel: [w446] -> w400
        tunnel: w404 -> [w447]
        tunnel: [w448] -> w399
        tunnel: w403 -> [w448]
        tunnel: w378 -> [w443]
        tunnel: w402 -> [w458]
        tunnel: w401 -> [w456]
        tunnel: [w456] -> w398
        tunnel: [w455] -> w397
        tunnel: w400 -> [w455]
        tunnel: [w454] -> w396
        tunnel: w399 -> [w454]
        tunnel: w398 -> [w463]
        tunnel: w397 -> [w465]
        tunnel: w396 -> [w464]
        tunnel: [w463] -> w395
        tunnel: [w462] -> w394
        tunnel: [w461] -> w393
        tunnel: w395 -> [w480]
        tunnel: w394 -> [w479]
        tunnel: w393 -> [_]
        tunnel: [w476] -> w392
        tunnel: w392 -> [w491]
        frame #0 {
          # "Arm Angle up"
          n143 = while {
            shift-right: [w418] -> w413
            shift-left: w415 -> [w417]
            shift-right: [w421] -> w412
            shift-left: w415 -> [w422]
            stop <- w424 stop-if-true
            n144 = call <vilib>:"Spark MAX Get Sensor Position.vi"("MotorControlDevRef in"=w422) -> ("Sensor Position"=w420:dbl, "MotorControlDevRef out"=w421:T6)  [unwired: 7 in, 2 out]
            n145 = Absolute Value(x=w420) -> (abs(x)=w416:dbl)
            n146 = call <vilib>:"WPI_MotorControlSetOutput.vi"("Output"=0.2 ("Left axis value"), "MotorControlDevRef"=w417) -> ("MotorControlDevRef"=w418:T6)  [unwired: 7 in, 2 out]
            n147 = Greater Or Equal?(x=w416, y=93.0) -> (x >= y?=w424:bool)
            n148 = local write "Angle Position"(w416) -> ()
          }
          n149 = call-poly <vilib>:"WPI_SolenoidSet.vi"("Value"=WPI_SolenoidValue."Reverse", "SolenoidDevRef"=w410) -> ()  [unwired: 8 in, 2 out]
        }
        frame #1 {
          # "Arm Angle Stop"
          # "Arm Tellescope out"
          n150 = while {
            shift-right: [w436] -> w432
            shift-left: w426 -> [w435]
            shift-right: [w439] -> w431
            shift-left: w427 -> [w440]
            stop <- w442 stop-if-true
            w434 = T15 0 items=["PercentOutput"=0, "Position"=1, "Velocity"=2, "Current"=3, "Follower"=5, "MotionProfile"=6, "MotionMagic"=7, "MotionProfileArc"=10, "Disabled"=15] ("Control Mode")
            n151 = call-poly <vilib>:"CTRE_Phoenix_CANcoder_GetPolymorphic.vi"("CTRE_CANcoder_DeviceRef"=w440) -> ("CTRE_CANcoder_DeviceRef"=w439:T12, "Position"=w438:dbl)  [unwired: 10 in, 3 out]
            n152 = Absolute Value(x=w438) -> (abs(x)=w433:dbl)
            n153 = call <vilib>:"CTRE_Phoenix_MotorControl_Set.vi"("Output"=0.35 ("Left axis value"), "Control Mode"=w434, "PhoenixMotorControlDevRef"=w435) -> ("PhoenixMotorControlDevRef"=w436:T6)  [unwired: 7 in, 1 out]
            n154 = local write "Arm Tellescope position"(w433) -> ()
            n155 = Greater Or Equal?(x=w433, y=1790.0) -> (x >= y?=w442:bool)
          }
          n156 = call <vilib>:"WPI_MotorControlSetOutput.vi"("Output"=0.0, "MotorControlDevRef"=w430) -> ("MotorControlDevRef"=w429:T6)  [unwired: 7 in, 2 out]
        }
        frame #2 {
          w445 = T15 0 items=["PercentOutput"=0, "Position"=1, "Velocity"=2, "Current"=3, "Follower"=5, "MotionProfile"=6, "MotionMagic"=7, "MotionProfileArc"=10, "Disabled"=15] ("Control Mode")
          w453 = T15 0 items=["PercentOutput"=0, "Position"=1, "Velocity"=2, "Current"=3, "Follower"=5, "MotionProfile"=6, "MotionMagic"=7, "MotionProfileArc"=10, "Disabled"=15] ("Control Mode")
          # "Arm Tellescope stop"
          # "Shoot"
          n157 = call <vilib>:"CTRE_Phoenix_MotorControl_Set.vi"("Output"=0.0, "Control Mode"=w445, "PhoenixMotorControlDevRef"=w447) -> ("PhoenixMotorControlDevRef"=w446:T6)  [unwired: 7 in, 1 out]
          n158 = Wait (ms)(milliseconds to wait=u32 1000) -> ()  [unwired: 1 out]
          n159 = call <vilib>:"CTRE_Phoenix_MotorControl_Set.vi"("Output"=0.3, "Control Mode"=w453, "PhoenixMotorControlDevRef"=w443) -> ("PhoenixMotorControlDevRef"=w450:T6)  [unwired: 7 in, 1 out]
        }
        frame #3 {
          w459 = T15 0 items=["PercentOutput"=0, "Position"=1, "Velocity"=2, "Current"=3, "Follower"=5, "MotionProfile"=6, "MotionMagic"=7, "MotionProfileArc"=10, "Disabled"=15] ("Control Mode")
          # "Stop Shooting"
          n160 = Wait (ms)(milliseconds to wait=u32 250) -> ()  [unwired: 1 out]
          n161 = call <vilib>:"CTRE_Phoenix_MotorControl_Set.vi"("Output"=0.0, "Control Mode"=w459, "PhoenixMotorControlDevRef"=w458) -> ()  [unwired: 7 in, 2 out]
        }
        frame #4 {
          # "Arm Tellescope back in"
          n162 = while {
            shift-right: [w469] -> w462
            shift-left: w465 -> [w468]
            shift-right: [w472] -> w461
            shift-left: w464 -> [w473]
            stop <- w475 stop-if-true
            w467 = T15 0 items=["PercentOutput"=0, "Position"=1, "Velocity"=2, "Current"=3, "Follower"=5, "MotionProfile"=6, "MotionMagic"=7, "MotionProfileArc"=10, "Disabled"=15] ("Control Mode")
            n163 = call-poly <vilib>:"CTRE_Phoenix_CANcoder_GetPolymorphic.vi"("CTRE_CANcoder_DeviceRef"=w473) -> ("CTRE_CANcoder_DeviceRef"=w472:T12, "Position"=w471:dbl)  [unwired: 10 in, 3 out]
            n164 = Absolute Value(x=w471) -> (abs(x)=w466:dbl)
            n165 = call <vilib>:"CTRE_Phoenix_MotorControl_Set.vi"("Output"=-0.3 ("Left axis value"), "Control Mode"=w467, "PhoenixMotorControlDevRef"=w468) -> ("PhoenixMotorControlDevRef"=w469:T6)  [unwired: 7 in, 1 out]
            n166 = Less Or Equal?(x=w466, y=30.0) -> (x <= y?=w475:bool)
            n167 = local write "Arm Tellescope position"(w466) -> ()
          }
        }
        frame #5 {
          w477 = T15 0 items=["PercentOutput"=0, "Position"=1, "Velocity"=2, "Current"=3, "Follower"=5, "MotionProfile"=6, "MotionMagic"=7, "MotionProfileArc"=10, "Disabled"=15] ("Control Mode")
          # "Arm Tellescope stop"
          # "Arm Angle down"
          n168 = while {
            shift-right: [w484] -> w476
            shift-left: w480 -> [w483]
            shift-right: [w486] -> _
            shift-left: w480 -> [w487]
            stop <- w489 stop-if-true
            n169 = call <vilib>:"Spark MAX Get Sensor Position.vi"("MotorControlDevRef in"=w487) -> ("Sensor Position"=w485:dbl, "MotorControlDevRef out"=w486:T6)  [unwired: 7 in, 2 out]
            n170 = Absolute Value(x=w485) -> (abs(x)=w481:dbl)
            n171 = call <vilib>:"WPI_MotorControlSetOutput.vi"("Output"=-0.15 ("Left axis value"), "MotorControlDevRef"=w483) -> ("MotorControlDevRef"=w484:T6)  [unwired: 7 in, 2 out]
            n172 = Less Or Equal?(x=w481, y=5.0) -> (x <= y?=w489:bool)
            n173 = local write "Angle Position"(w481) -> ()
          }
          n174 = call <vilib>:"CTRE_Phoenix_MotorControl_Set.vi"("Output"=0.0, "Control Mode"=w477, "PhoenixMotorControlDevRef"=w479) -> ()  [unwired: 7 in, 2 out]
        }
        frame #6 {
          # "Arm Angle Stop"
          n175 = call <vilib>:"WPI_MotorControlSetOutput.vi"("Output"=0.0, "MotorControlDevRef"=w491) -> ()  [unwired: 7 in, 3 out]
        }
      }
    }
    frame "Charge Station Only" {
      # "Move straight out"
      n176 = call <vilib>:"CTRE_Phoenix_MotorControl_RefNumRegistryGet.vi"("refnum name"="Talon FX Left Encoder") -> ("PhoenixMotorControlDevRef"=w495:T6)  [unwired: 9 in, 1 out]
      n177 = call <vilib>:"CTRE_Phoenix_MotorControl_RefNumRegistryGet.vi"("refnum name"="Talon FX Right  Encoder") -> ("PhoenixMotorControlDevRef"=w496:T6)  [unwired: 9 in, 1 out]
      n178 = call <vilib>:"WPI_SolenoidRefNum Registry Get.vi"("refnum name"="Breaks") -> ("SolenoidDevRef"=w492:T13)  [unwired: 9 in, 1 out]
      n179 = call <vilib>:"WPI_RobotDriveRefNum Registry Get.vi"("refnum name"="Tank Drive Motors") -> ("RobotDriveDevRef"=w499:T11)  [unwired: 9 in, 1 out]
      n180 = flat-sequence {
        tunnel: w499 -> [w512]
        tunnel: [w511] -> w503
        tunnel: [w510] -> w502
        tunnel: [w509] -> w501
        tunnel: w495 -> [w508]
        tunnel: w496 -> [w507]
        tunnel: w492 -> [w505]
        tunnel: [w504] -> w493
        tunnel: w503 -> [w537]
        tunnel: w502 -> [w533]
        tunnel: w501 -> [w536]
        tunnel: w493 -> [w532]
        frame #0 {
          n181 = while {
            shift-right: [w527] -> w511
            shift-left: w512 -> [w530]
            shift-right: [w525] -> w510
            shift-left: w508 -> [w528]
            shift-right: [w526] -> w509
            shift-left: w507 -> [w529]
            stop <- w522 stop-if-true
            w519 = 2048 ("y")
            w521 = 0.4 ("Left axis value")
            # "Invert axis to flip back wheels\nnegative"
            n182 = call-poly <vilib>:"CTRE_Phoenix_MotorController_Get_TalonFX.vi"("PhoenixMotorControlDevRef"=w528) -> ("PhoenixMotorControlDevRef"=w525:T6, "Position (Raw Sensor Units)"=w524:i32)  [unwired: 11 in, 2 out]
            n183 = call-poly <vilib>:"CTRE_Phoenix_MotorController_Get_TalonFX.vi"("PhoenixMotorControlDevRef"=w529) -> ("PhoenixMotorControlDevRef"=w526:T6, "Position (Raw Sensor Units)"=w523:i32)  [unwired: 11 in, 2 out]
            n184 = Absolute Value(x=w523) -> (abs(x)=w517:i32)
            n185 = Absolute Value(x=w524) -> (abs(x)=w518:i32)
            n186 = call <vilib>:"WPI_RobotDriveTankDrive.vi"("Right axis value"=w521, "Left axis value"=w521, "RobotDriveDevRef"=w530) -> ("RobotDriveDevRef"=w527:T11)  [unwired: 6 in, 2 out]
            n187 = Divide(x=w518, y=w519) -> (x/y=w516:dbl)
            n188 = Divide(x=w517, y=w519) -> (x/y=w515:dbl)
            n189 = Round To Nearest(number=w516) -> (nearest integer value=w513:dbl)
            n190 = Round To Nearest(number=w515) -> (nearest integer value=w514:dbl)
            n191 = Subtract(x=w513, y=w514) -> ()  [unwired: 1 out]
            n192 = Greater Or Equal?(x=w513, y=75) -> (x >= y?=w522:bool)
            n193 = local write "Talon Encoder Values"(w513) -> ()
          }
          n194 = call-poly <vilib>:"WPI_SolenoidSet.vi"("Value"=WPI_SolenoidValue."Reverse", "SolenoidDevRef"=w505) -> ("SolenoidDevRef"=w504:T13)  [unwired: 8 in, 1 out]
        }
        frame #1 {
          w538 = 0.0
          n195 = call <vilib>:"CTRE_Phoenix_MotorControl_SetSelectedSensorPosition.vi"("New Sensor Position"=0, "PhoenixMotorControlDevRef"=w536) -> ()  [unwired: 8 in, 2 out]
          n196 = call <vilib>:"CTRE_Phoenix_MotorControl_SetSelectedSensorPosition.vi"("New Sensor Position"=0, "PhoenixMotorControlDevRef"=w533) -> ()  [unwired: 8 in, 2 out]
          n197 = call <vilib>:"WPI_RobotDriveTankDrive.vi"("Right axis value"=w538, "Left axis value"=w538, "RobotDriveDevRef"=w537) -> ()  [unwired: 6 in, 3 out]
          n198 = call-poly <vilib>:"WPI_SolenoidSet.vi"("Value"=WPI_SolenoidValue."Forward", "SolenoidDevRef"=w532) -> ()  [unwired: 8 in, 2 out]
        }
      }
    }
    frame "Your Turn" {
    }
  }
